vi "TDMSAdv overwriteComment.vi"(7 "timeStamp":string="2019/01/16 09:44:55.1", 8 "error in (no error)":errorcluster, 9 "newComment":string, 10 "file path":path, 11 "TDMSAdv in":refnum<class "TDMSAdv.lvclass">) -> (0 "error out":errorcluster, 3 "TDMSAdv out":refnum<class "TDMSAdv.lvclass">)   [LabVIEW 2018, in "TDMSAdv.lvclass"]
uses:
  TDMSAdv.lvclass
  TDMSAdv.lvclass/TDMSAdv.ctl
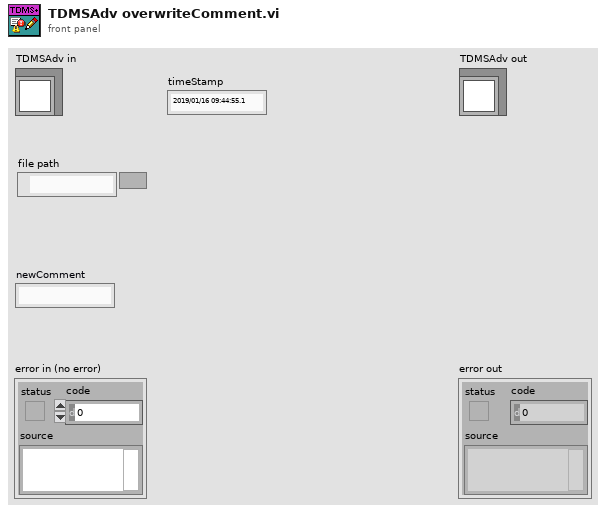
[diagram p1: front panel]
types:
  T1 = enum16{"open", "open or create", "create or replace", "create", "open (read-only)"}
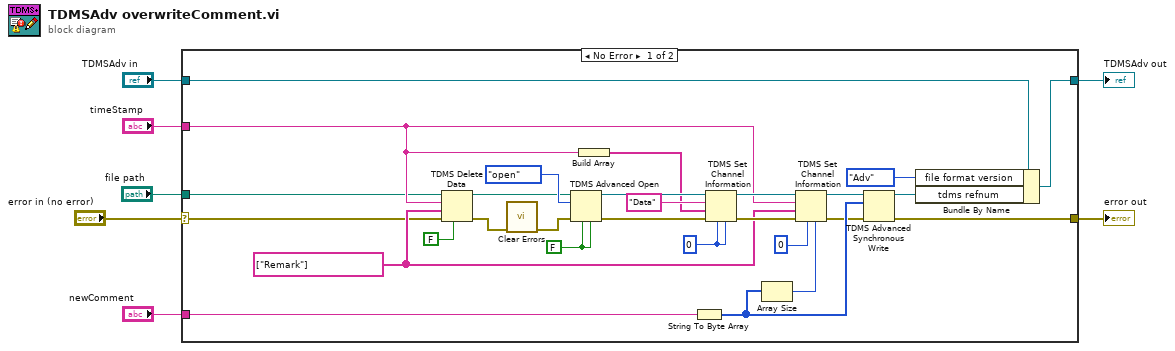
[diagram p0: block diagram]
diagram:
  n1 = case shown="No Error" "error in (no error)" {
    selector: "error in (no error)" -> [w8 w37]
    tunnel: [w14 w37] -> w6
    tunnel: [w13 w36] -> w4
    tunnel: "TDMSAdv in" -> [w16 w36]
    tunnel: "timeStamp" -> [w19 _]
    tunnel: "newComment" -> [w17 _]
    tunnel: "file path" -> [w9 _]
    frame No Error {
      w32 = u8 0 ("data type")
      w34 = FALSE ("disable buffering? (T)")
      w18 = string[] ["Remark"] ("channel name(s)")
      n2 = TDMS Delete Data(6:FALSE ("keep empty group/channel? (T)"), 8:w8, 9:w18, 10:w19, 11:w9) -> (0:w11:errorcluster, 3:w20:path)  [unwired: 2 in]
      n3 = call <vilib>:"Clear Errors.vi"("error in (no error)"=w11) -> ("error out"=w10:errorcluster)  [unwired: 5 in, 1 out]
      n4 = TDMS Advanced Open(4:w34, 6:w34, 8:w10, 10:T1."open" ("operation (0:open)"), 11:w20) -> (0:w30:errorcluster, 3:w31:refnum<k34>)  [unwired: 1 out]
      n5 = Build Array(w19) -> (w22:string[])
      n6 = String To Byte Array(string=w17) -> (unsigned byte array=w27:u8[])
      n7 = TDMS Set Channel Information(4:w32, 6:w32, 8:w30, 9:w22, 10:"Data" ("group name (Untitled)"), 11:w31) -> (0:w21:errorcluster, 3:w23:refnum<k34>)  [unwired: 1 in]
      n8 = Array Size(array=w27) -> (size(s)=w28:i32)
      n9 = TDMS Set Channel Information(4:w28, 6:u8 0, 8:w21, 9:w18, 10:w19, 11:w23) -> (0:w25:errorcluster, 3:w26:refnum<k34>)  [unwired: 1 in]
      n10 = TDMS Advanced Synchronous Write(8:w25, 10:w27, 11:w26) -> (0:w14:errorcluster, 3:w15:refnum<k34>)
      n11 = Bundle By Name(cluster=w16, "file format version"=enum16{"1.0", "2.0", "Adv"}."Adv", "tdms refnum"=w15) -> (w13:refnum<class "TDMSAdv.lvclass">)
    }
    frame Error {
    }
  }
  "error out" <- w6
  "TDMSAdv out" <- w4
